vi "PuTTY.vi"() -> ()   [LabVIEW 2010]
panel:
  in  "Command(s) to Execute":string="ssh almaproc@10.192.1.123 'python /users/almaproc/scripts/testCanMonitor -a test-abm -c 1'"
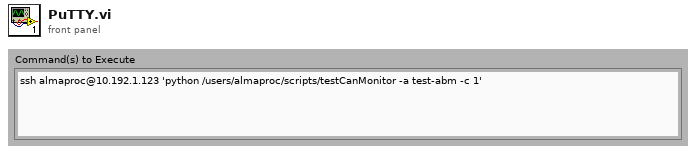
[diagram p1: front panel]
types:
  T1 = enum32{"invalid app kind", "Development System", "Run Time System", "Student Edition", "Embedded LabVIEW", "Evaluation", "Custom"}
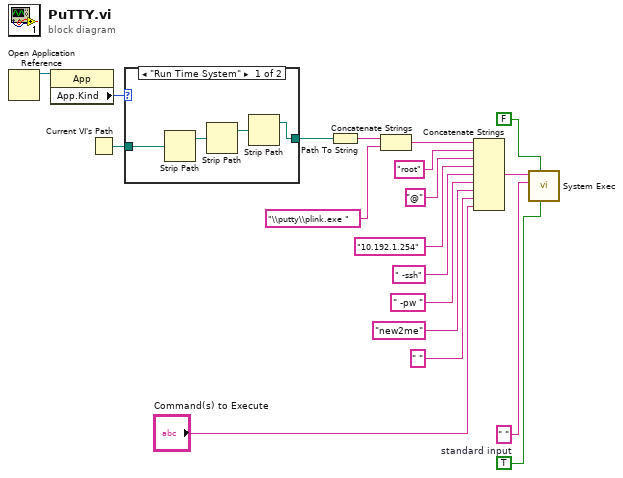
[diagram p0: block diagram]
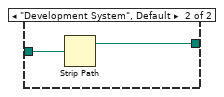
[diagram p2: hidden frame]
diagram:
  w19 = " "  # standard input
  n1 = Open Application Reference() -> (3:w11:refnum<vi>)  [unwired: 4 in, 1 out]
  n2 = property class="App"(reference=w11) -> ("App.Kind"=w10:T1)  [unwired: 1 in, 2 out]
  n3 = Current VI's Path() -> (path=w9:path)
  n4 = case shown="\"Run Time System\"" w10 {
    tunnel: w9 -> [w20 w25]
    tunnel: [w21 w24] -> w8
    frame "Run Time System" {
      n5 = Strip Path(path=w20) -> (stripped path=w22:path)  [unwired: 1 out]
      n6 = Strip Path(path=w22) -> (stripped path=w23:path)  [unwired: 1 out]
      n7 = Strip Path(path=w23) -> (stripped path=w21:path)  [unwired: 1 out]
    }
    frame "Development System", Default {
      n8 = Strip Path(path=w25) -> (stripped path=w24:path)  [unwired: 1 out]
    }
  }
  n9 = Path To String(path=w8) -> (string=w5:string)
  n10 = Concatenate Strings(w5, "\\putty\\plink.exe " ("command line")) -> (w6:string)
  n11 = Concatenate Strings(w6, "root" ("Username"), "@" ("string"), "10.192.1.254" ("Host"), " -ssh", " -pw " ("string"), "new2me" ("Password"), " " ("string"), "Command(s) to Execute") -> (w12:string)
  n12 = call <vilib>:"System Exec.vi"("run minimized? (F)"=TRUE ("Hide DOS\nWindow?"), "wait until completion? (T)"=FALSE, "standard input"=w19, "command line"=w12) -> ()  [unwired: 2 in, 6 out]
